vi "Variant to ADS Type Byte Stream.vi"(7 "Type Name":string, 8 "error in (no error)":errorcluster, 10 "Value":variant, 11 "TwinCAT ADS in":refnum<class "TwinCAT ADS.lvclass">) -> (0 "error out":errorcluster, 2 "Byte Stream":u8[](array[numeric]), 3 "TwinCAT ADS out":refnum<class "TwinCAT ADS.lvclass">)   [LabVIEW 2018, in "TwinCAT ADS.lvclass"]
uses:
  TwinCAT ADS.lvclass
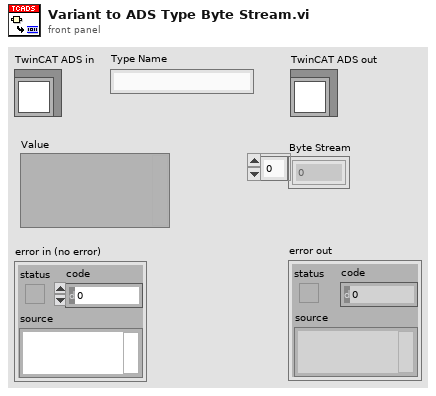
[diagram p1: front panel]
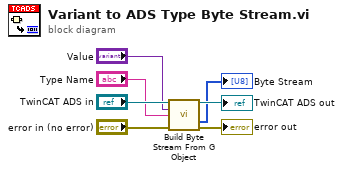
[diagram p0: block diagram]
diagram:
  n1 = call "Build Byte Stream From G Object.vi"("TwinCAT ADS in"="TwinCAT ADS in", "Value"="Value", "Type Name"="Type Name", "error in (no error)"="error in (no error)") -> ("TwinCAT ADS out"=→"TwinCAT ADS out":refnum<class "TwinCAT ADS.lvclass">, "Byte Stream out"=→"Byte Stream":u8[], "error out"=→"error out":errorcluster)  [unwired: 9 in]
